vi "AI one shot test.vi"() -> ()   [LabVIEW 2019]
uses:
  <vilib>/DAQmx/read.llb/DAQmx Read (Analog 2D DBL NChan NSamp).vi
  <vilib>/Analysis/baseanly.llb/Mean (DBL).vi
  <vilib>/DAQmx/create/channels.llb/DAQmx Create Channel (AI-Voltage-Basic).vi
  <vilib>/DAQmx/configure/timing.llb/DAQmx Timing (Sample Clock).vi
  <vilib>/DAQmx/miscellaneous.llb/DAQmx Fill In Error Info.vi
  <resource>/objmgr/daqmx.rc
  <vilib>/Analysis/NI_AALBase.lvlib
panel:
  out "error out 2":errorcluster
  out "AI voltage":dbl[](array[numeric])
  out "millisecond timer value":u32
  out "x-y":u32 format="%.6f"
  in  "sample mode":i32(ring)=10123 items=["Finite Samples"=10178, "Continuous Samples"=10123, "Hardware Timed Single Point"=12522]
  in  "Data rate (hz)":dbl=500.0
  in  "error in":errorcluster
  out "error out":errorcluster
  out "Data":dbl[](array[numeric]) format="%#.5g"
  in  "samples per channel":i32=10 min=1 step=1
  in  "stop":bool
  out "Waveform Chart":dbl[][](graph)
  # "—The progammable-gain amplifier provides input gains of 1, 2, 4, 5, 8, 10, 16, or 20"
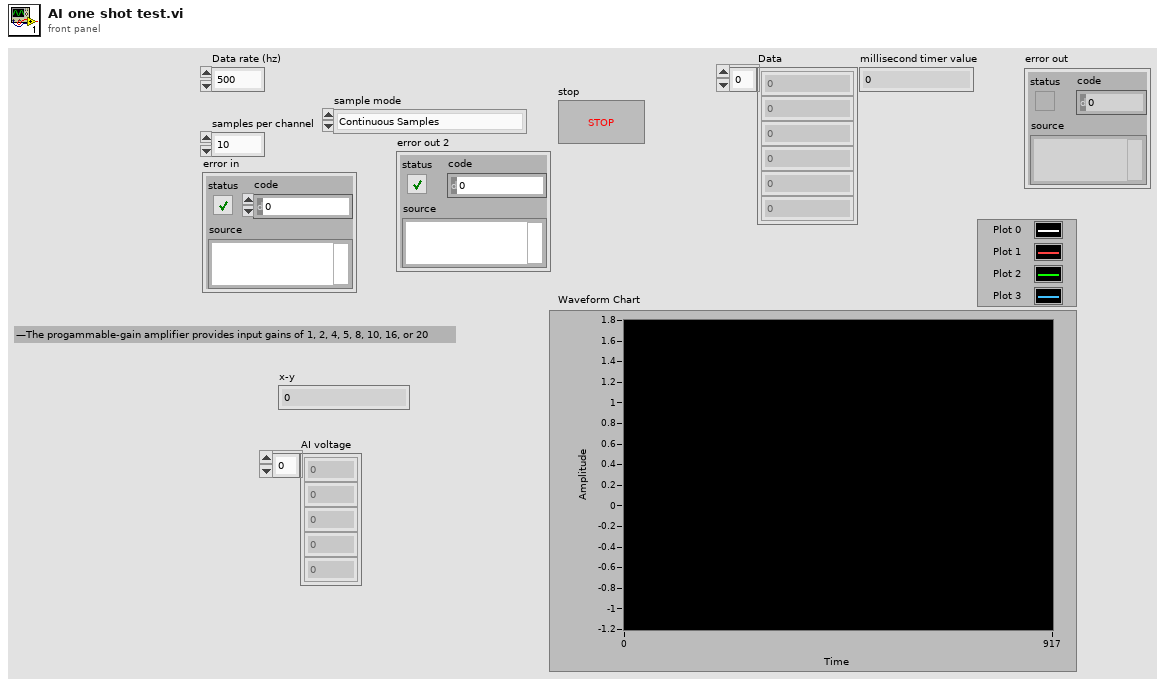
[diagram p1: front panel]
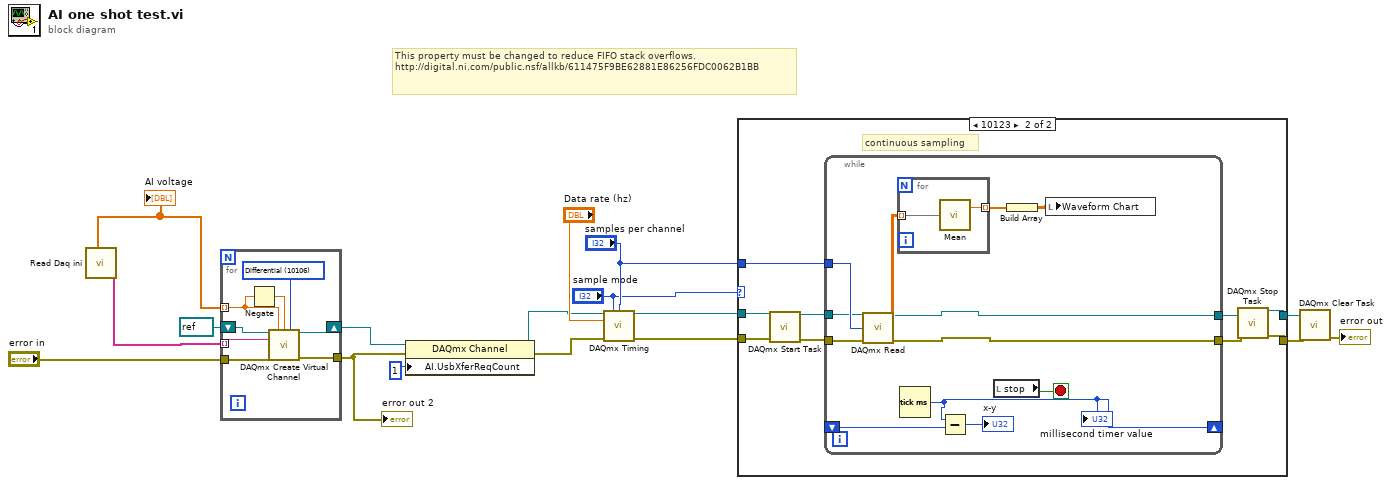
[diagram p0: block diagram]
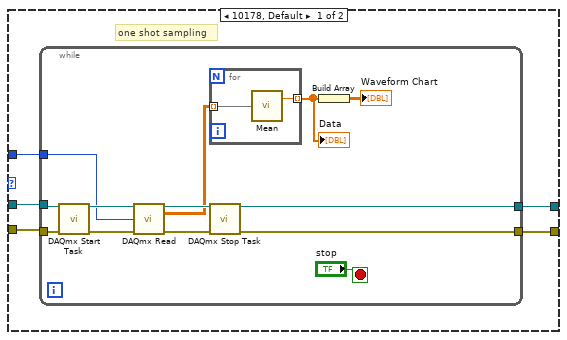
[diagram p2: hidden frame]
diagram:
  # "This property must be changed to reduce FIFO stack overflows.\nhttp://digital.ni.com/public.nsf/allkb/611475F9BE62881E86256FDC0062B1BB"
  n1 = call "Read Daq ini.vi"() -> ("AI Channels"=w3:string[], "AI voltage"=w1:dbl[])  [unwired: 3 in, 7 out]
  "AI voltage" <- w1
  n2 = for {
    tunnel: [w25] -> w14
    tunnel: w3 -> [w23] mode=indexing
    tunnel: "error in" -> [w22]
    shift-right: [w24] -> w11
    shift-left: refnum<k21> refnum ("task out") -> [w21]
    tunnel: w1 -> [w20] mode=indexing
    w18 = 10106 items=["default"=-1, "RSE"=10083, "NRSE"=10078, "Differential"=10106, "Pseudodifferential"=12529] ("input terminal configuration")
    n3 = Negate(x=w20) -> (-x=w19:dbl)
    n4 = call-poly <vilib>:"DAQmx Create Virtual Channel.vi"("task in"=w21, "maximum value"=w20, "minimum value"=w19, "input terminal configuration"=w18, "physical channels"=w23, "error in"=w22) -> ("task out"=w24:refnum<k21>, "error out"=w25:errorcluster)  [unwired: 8 in]
  }
  "error out 2" <- w14
  n5 = property class="DAQmx Channel"(reference=w11, error in=w14, "AI.UsbXferReqCount"=u32 1) -> (reference out=w7:refnum<k21>, error out=w9:errorcluster)
  n6 = call-poly <vilib>:"DAQmx Timing.vi"("task/channels in"=w7, "sample mode"="sample mode", "samples per channel"="samples per channel", "rate"="Data rate (hz)", "error in"=w9) -> ("task out"=w6:refnum<k21>, "error out"=w8:errorcluster)  [unwired: 9 in]
  n7 = case shown="10123" "sample mode" {
    tunnel: [w30 w50] -> w16
    tunnel: [w29 w52] -> w15
    tunnel: w8 -> [w28 w48]
    tunnel: w6 -> [w27 w49]
    tunnel: "samples per channel" -> [w26 w54]
    frame 10178, Default {
      # "one shot sampling"
      n8 = while {
        tunnel: w27 -> [w32]
        tunnel: w28 -> [w31]
        tunnel: [w40] -> w30
        tunnel: [w39] -> w29
        tunnel: w26 -> [w33]
        stop <- "stop" stop-if-true
        n9 = call <vilib>:"DAQmx Start Task.vi"("task/channels in"=w32, "error in"=w31) -> ("task out"=w42:refnum<k21>, "error out"=w43:errorcluster)  [unwired: 12 in]
        n10 = call-poly <vilib>:"DAQmx Read.vi"("task/channels in"=w42, "number of samples per channel"=w33, "error in"=w43) -> ("task out"=w41:refnum<k21>, "data"=w37:dbl[][], "error out"=w36:errorcluster)  [unwired: 10 in]
        n11 = for {
          tunnel: w37 -> [w45] mode=indexing
          tunnel: [w44] -> w34 mode=indexing
          n12 = call-poly <vilib>:"Mean.vi"("X"=w45) -> ("mean"=w44:dbl)  [unwired: 1 out]
        }
        "Data" <- w34
        n13 = call <vilib>:"DAQmx Stop Task.vi"("task/channels in"=w41, "error in"=w36) -> ("task out"=w39:refnum<k21>, "error out"=w40:errorcluster)  [unwired: 12 in]
        n14 = Build Array(w34) -> (→"Waveform Chart":dbl[][])
      }
    }
    frame 10123 {
      # "continuous sampling"
      n15 = call <vilib>:"DAQmx Start Task.vi"("task/channels in"=w49, "error in"=w48) -> ("task out"=w47:refnum<k21>, "error out"=w46:errorcluster)  [unwired: 12 in]
      n16 = while {
        tunnel: w46 -> [w63]
        tunnel: [w61] -> w51
        tunnel: [w62] -> w53
        tunnel: w54 -> [w64]
        tunnel: w47 -> [w60]
        shift-right: [w56] -> _
        shift-left: _ -> [w57]
        stop <- w59 stop-if-true
        n17 = call-poly <vilib>:"DAQmx Read.vi"("task/channels in"=w60, "number of samples per channel"=w64, "error in"=w63) -> ("task out"=w62:refnum<k21>, "data"=w66:dbl[][], "error out"=w61:errorcluster)  [unwired: 10 in]
        n18 = for {
          tunnel: w66 -> [w68] mode=indexing
          tunnel: [w67] -> w65 mode=indexing
          n19 = call-poly <vilib>:"Mean.vi"("X"=w68) -> ("mean"=w67:dbl)  [unwired: 1 out]
        }
        n20 = Tick Count (ms)() -> (millisecond timer value=w56:u32)
        "millisecond timer value" <- w56
        n21 = Subtract(x=w56, y=w57) -> (x-y=→"x-y":u32)
        n22 = local read "stop"() -> (w59:bool)
        n23 = Build Array(w65) -> (w58:dbl[][])
        n24 = local write "Waveform Chart"(w58) -> ()
      }
      n25 = call <vilib>:"DAQmx Stop Task.vi"("task/channels in"=w53, "error in"=w51) -> ("task out"=w52:refnum<k21>, "error out"=w50:errorcluster)  [unwired: 12 in]
    }
  }
  n26 = call <vilib>:"DAQmx Clear Task.vi"("task in"=w15, "error in"=w16) -> ("error out"=→"error out":errorcluster)  [unwired: 13 in]
